vi "timestamp analysis(SubVI).vi"(8 "newer than 240815":bool, 10 "first row":dbl[](array[numeric]), 11 "start pos correct":dbl) -> (1 "Numeric":dbl, 2 "Array":dbl[](array[numeric]), 3 "Array 2":dbl[](array[numeric]))   [LabVIEW 2024]
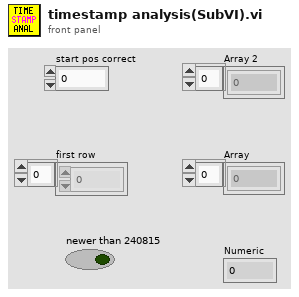
[diagram p1: front panel]
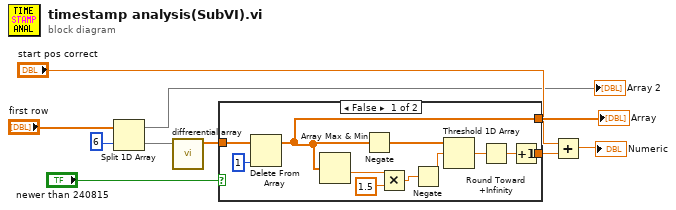
[diagram p0: block diagram]
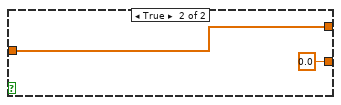
[diagram p2: hidden frame]
diagram:
  n1 = Split 1D Array(array="first row", index=6) -> (first subarray=→"Array 2":dbl[], second subarray=w5:dbl[])
  n2 = call "diffrerential array.vi"("Array in"=w5) -> ("Array"=w1:dbl[])  [unwired: 10 in]
  n3 = case shown="False" "newer than 240815" {
    tunnel: [w21 0.0] -> w10
    tunnel: [w20 w22] -> w9
    tunnel: w1 -> [w11 w22]
    frame False {
      n4 = Delete From Array(array=w11, index=1) -> (array with subset deleted=w20:dbl[])  [unwired: 1 in, 1 out]
      n5 = Array Max & Min(array=w20) -> (min value=w13:dbl)  [unwired: 3 out]
      n6 = Negate(x=w20) -> (-x=w18:dbl[])
      n7 = Multiply(x=w13, y=1.5) -> (x*y=w15:dbl)
      n8 = Negate(x=w15) -> (-x=w19:dbl)
      n9 = Threshold 1D Array(2:w19, 3:w18) -> (0:w16:dbl)  [unwired: 1 in]
      n10 = Round Toward +Infinity(x=w16) -> (ceil(x): smallest int >= x=w17:dbl)
      n11 = Increment(x=w17) -> (x+1=w21:dbl)
    }
    frame True {
    }
  }
  "Array" <- w9
  n12 = Add(x="start pos correct", y=w10) -> (x+y=→"Numeric":dbl)
